vi "checkDisplacementST.vi"(8 "error in (no error)":errorcluster, 11 "Model in":refnum<class "Model.lvclass">) -> (0 "error out":errorcluster, 2 "reachedDisplacementTriggerIsTrue":bool, 3 "Model out":refnum<class "Model.lvclass">)   [LabVIEW 2015, in "Model.lvclass"]
uses:
  Model.lvclass
  Model.lvclass/Model.ctl
  <userlib>/Common/Devices/DistanceGauge/DistanceGauge/DistanceGauge.lvclass/DistanceGauge.ctl
  <userlib>/Common/Devices/DistanceGauge/DistanceGauge/DistanceGauge.lvclass
  ApplicationElements/SystemController/SystemController.lvclass
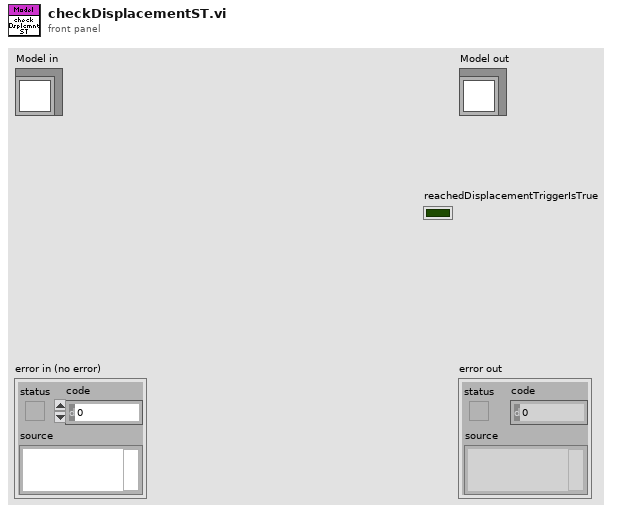
[diagram p1: front panel]
types:
  T1 = typedef "DistanceGauge.lvlib/Distance Data.ctl" = cluster{"Distance Measured 1":dbl[unit], "Distance Measured 2":dbl[unit]}
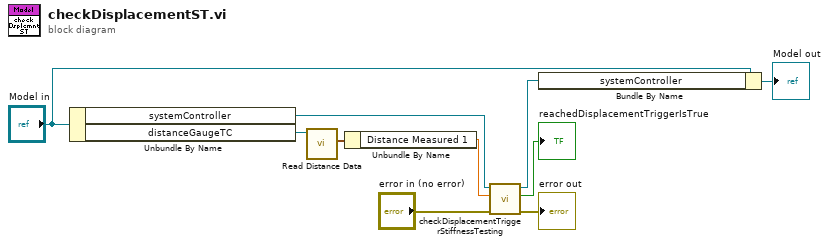
[diagram p0: block diagram]
diagram:
  n1 = Unbundle By Name("Model in") -> ("systemController"=w10:refnum<class "SystemController.lvclass">, "distanceGaugeTC"=w9:refnum<class "DistanceGaugeTC.lvclass">)
  n2 = call <userlib>:"Read Distance Data.vi"("DistanceGauge in"=w9) -> ("Distance Data"=w8:T1)  [unwired: 9 in, 1 out]
  n3 = Unbundle By Name(w8) -> ("Distance Measured 1"=w7:dbl[unit])
  n4 = call "checkDisplacementTriggerStiffnessTesting.vi"("error in (no error)"="error in (no error)", "Distance Measured"=w7, "SystemController in"=w10) -> ("error out"=→"error out":errorcluster, "displacementTriggerReached"=→"reachedDisplacementTriggerIsTrue":bool, "SystemController out"=w6:refnum<class "SystemController.lvclass">)  [unwired: 6 in]
  n5 = Bundle By Name(cluster="Model in", "systemController"=w6) -> (→"Model out":refnum<class "Model.lvclass">)
